vi "BallCacher.vi"() -> ()   [LabVIEW 2012]
doc: "This VI demonstrates how to control the Robotics Starter Kit 2.0 robot. It is deployed to an sbRIO-9632, then run on the Real-Time controller."
uses:
  <vilib>/Platform/TimedLoop/XDataNode/timing_clust.ctl
  <vilib>/Platform/TimedLoop/XDataNode/nitl_modes.ctl
  <vilib>/Platform/TimedLoop/XDataNode/wakeup.ctl
  <vilib>/robotics/Starter Kit/2.0/9632 Host Interface/NI_Robotics_Starter Kit Host_9632_2.0.lvclass
  <vilib>/Utility/AngleManip/Degrees to Radians (Scalar DBL).vi
  <vilib>/robotics/Steering/Steering Frame/Apply Steering Frame Velocity to Motors.vi
  <vilib>/Platform/TimedLoop/XDataNode/XDataNode.xnode
  <vilib>/Utility/AngleManip/NI_AngleManipulation.lvlib
  <vilib>/Platform/TimedLoop/XDataNode/XDNodeRunTimeDep.lvlib
  <vilib>/robotics/Utilities/Scan Angles/NI_Robotics_Scan Angles.lvlib
  <vilib>/robotics/Starter Kit/2.0/NI_Robotics_Starter Kit Host_2.0.lvlib
  <vilib>/robotics/Steering/Steering Frame/NI_Robotics_Steering Frame.lvclass
  <vilib>/robotics/Starter Kit/Host Interface/NI_Robotics_Starter Kit Host.lvclass
panel:
  in  "Tank1":dbl[](array[numeric])=[1.0, 1.0]
  in  "Tank2":dbl[](array[numeric])=[50.0, 50.0]
  out "Sensor Data":cluster{"angles (deg)":dbl[], "distances":dbl[]}(graph)
  in  "stop":bool
  # "This VI demonstrates how to control the Robotics Starter Kit 2.0 robot. It is deployed to an sbRIO-9632, then run on the Real-Time controller.\n\nInstructions:\n\n1. Set the \"MOTORS\" switch off, then set the \"MASTER\" switch on.  Make sure the robot is connected to the network.\n\n2. Run this VI.  The VI will deploy, and the robot's sensor will start panning left and right.  Accept any prompts to save VIs before deploying.\n\n3. Disconnect the robot from the network so it is no longer tethered.\n\n4. Move the robot to a clear area, then set the \"MOTORS\" switch on.  It will move and avoid obstacles.\n\n5. Set the \"MOTORS\" switch off to shut off power to the motors.\n\n6. Set the \"MASTER\" switch off to shut off power to the entire robot.  You will need to repeat steps 1 through 4 to redeploy after shutting off power*.\n\n*View Starter Kit 2.0 Readme.html for instructions on how to automatically run this VI on startup."
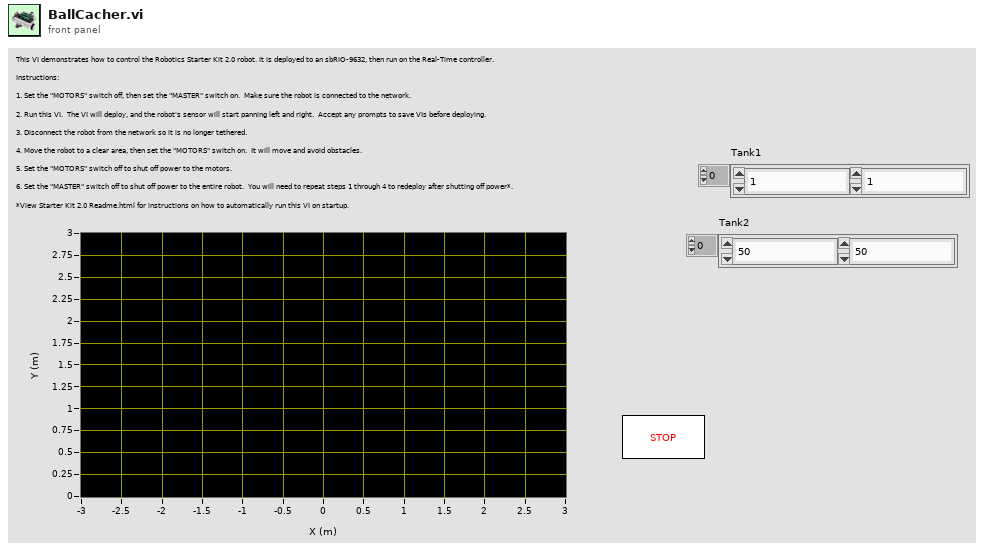
[diagram p1: front panel]
types:
  T1 = typedef "XDNodeRunTimeDep.lvlib/timing_clust.ctl" = cluster{"Expected End [f-1]":u64, "Actual End [f-1]":u64, "Finished Late? [f-1]":bool, "Expected End [i-1]":u64, "Actual End [i-1]":u64, "Finished Late? [i-1]":bool, "Expected Start [i]":u64, "Actual Start [i]":u64, "Expected Start [f]":u64, "Actual Start [f]":u64, "Source Name":string, "Structure Name":string, "Period":i64, "Deadline":i64, "Offset":i64, "Start":i64, "Priority":i32, "Timeout":i32, "Mode":T2, "Wakeup Reason":T3, "Error":errorcluster, "Source Type":string, "Secondary Source Type":string, "Global End Time":u64, "Global Start Time":u64, "Frame Duration":u64, "Iteration Duration":u64, "Assigned CPU":i32, "I/O Scan Engine Mode":u32}
  T2 = typedef "XDNodeRunTimeDep.lvlib/nitl_modes.ctl" = enum32{"No Change", "Process missed periods, maintain original phase", "Discard missed periods, maintain original phase", "Process missed periods, ignore original phase", "Discard missed periods, ignore original phase"}
  T3 = typedef "XDNodeRunTimeDep.lvlib/wakeup.ctl" = enum32{"Normal", "Aborted", "Asynchronous wakeup", "Timing source error", "Timed loop error", "Timeout"}
  T4 = typedef "NI_Robotics_Scan Angles.lvlib/Scan Angle Data.ctl" = cluster{"angles":dbl[], "distances":dbl[], "current index":i32, "previous index":i32}
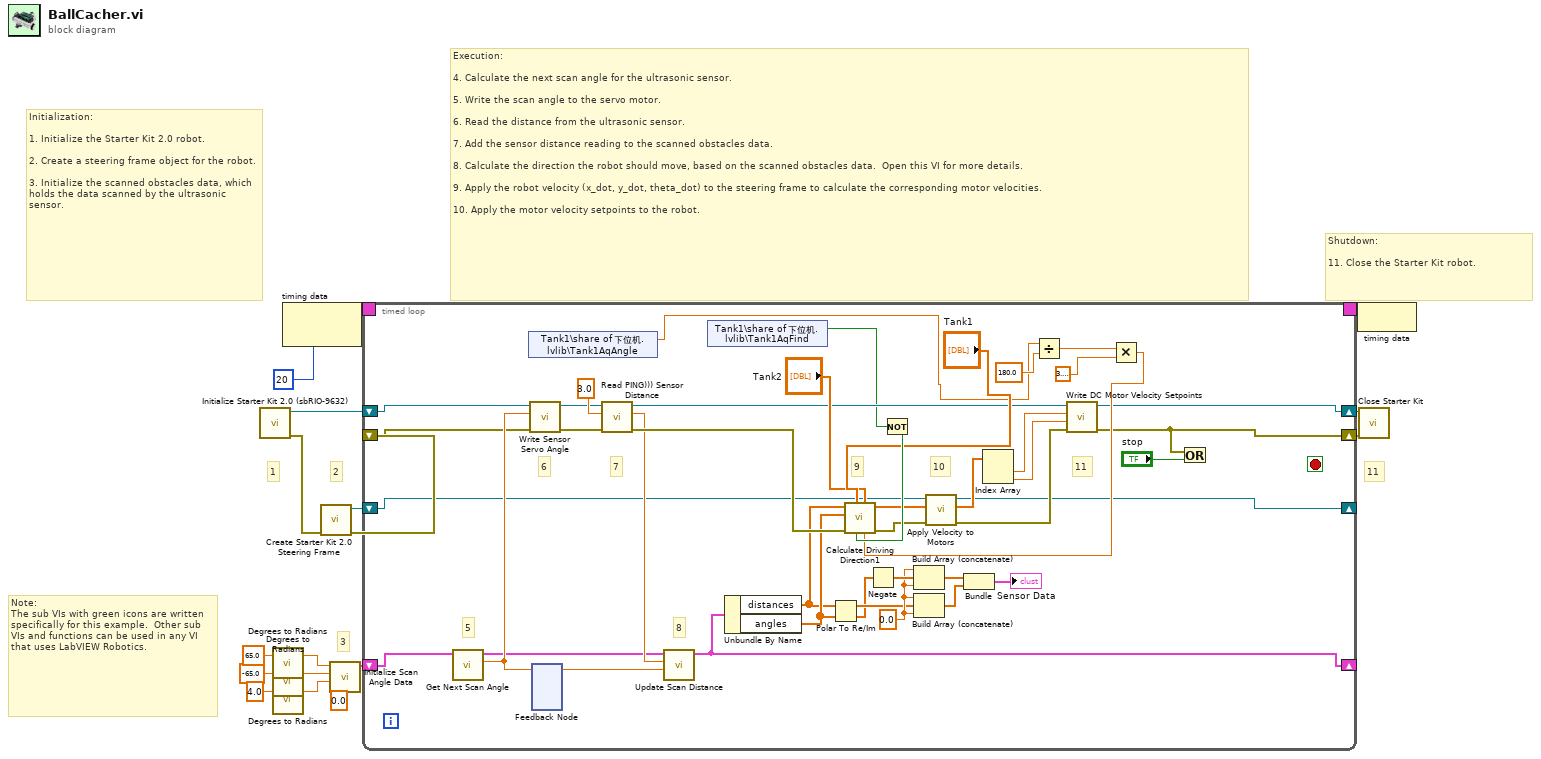
[diagram p0: block diagram]
diagram:
  # "11"
  # "Shutdown:\n\n11. Close the Starter Kit robot."
  # "Execution:\n\n4. Calculate the next scan angle for the ultrasonic sensor.\n\n5. Write the scan angle to the servo motor.\n\n6. Read the distance from the ultrasonic sensor.\n\n7. Add the sensor distance reading to the scanned obstacles data.\n\n8. Calculate the direction the robot should move, based on the scanned obstacles data.  Open this VI for more details.\n\n9. Apply the robot velocity (x_dot, y_dot, theta_dot) to the steering frame to calculate the corresponding motor velocities.\n\n10. Apply the motor velocity setpoints to the robot."
  # "3"
  # "2"
  # "1"
  # "Initialization:\n\n1. Initialize the Starter Kit 2.0 robot.\n\n2. Create a steering frame object for the robot.\n\n3. Initialize the scanned obstacles data, which holds the data scanned by the ultrasonic sensor."
  # "Note:\nThe sub VIs with green icons are written specifically for this example.  Other sub VIs and functions can be used in any VI that uses LabVIEW Robotics."
  n1 = call <vilib>:"Initialize Starter Kit 2.0 (sbRIO-9632).vi"() -> ("error out"=w1:errorcluster, "FPGA starter kit host 2.0 out"=w2:refnum<class "NI_Robotics_Starter Kit Host_9632_2.0.lvclass">)  [unwired: 10 in]
  n2 = call-poly <vilib>:"Degrees to Radians.vi"("angle (deg)"=65.0 ("max angle")) -> ("angle (rad)"=w12:dbl)  [unwired: 2 in]
  n3 = call-poly <vilib>:"Degrees to Radians.vi"("angle (deg)"=-65.0 ("min angle")) -> ("angle (rad)"=w8:dbl)  [unwired: 2 in]
  n4 = call-poly <vilib>:"Degrees to Radians.vi"("angle (deg)"=4.0 ("scan angle")) -> ("angle (rad)"=w9:dbl)  [unwired: 2 in]
  n5 = node-c288(i64 20 ("Period")) -> (w17:T1)
  n6 = call <vilib>:"Create Starter Kit 2.0 Steering Frame.vi"("error in (no error)"=w1) -> ("error out"=w5:errorcluster, "starter kit differential steering frame"=w6:refnum<class "NI_Robotics_Differential Steering Frame.lvclass">)  [unwired: 9 in]
  n7 = call <vilib>:"Initialize Scan Angle Data.vi"("initial angle (0)"=0.0, "scan angle"=w9, "min angle"=w8, "max angle"=w12) -> ("scan angles"=w14:T4)  [unwired: 6 in, 1 out]
  n8 = timed-loop {
    shift-right: [w20] -> _
    shift-left: w14 -> [w27]
    timing: w17 -> [_]
    timing-out: [_] -> w16
    shift-right: [w22] -> w3
    shift-left: w5 -> [w25]
    shift-right: [w23] -> w4
    shift-left: w2 -> [w24]
    shift-right: [w21] -> _
    shift-left: w6 -> [w26]
    stop <- _ stop-if-true
    w44 = 0.0 ("element")
    # "7"
    # "6"
    # "11"
    # "10"
    # "9"
    # "8"
    # "5"
    n9 = call <vilib>:"Get Next Scan Angle.vi"("scan angles in"=w27) -> ("new angle"=w32:dbl, "scan angles out"=w29:T4)  [unwired: 9 in]
    n10 = shared-variable "Tank1\\share of 下位机.lvlib\\Tank1AqAngle"() -> (w18:dbl)  [unwired: 1 in, 1 out]
    n11 = call <vilib>:"Write Sensor Servo Angle.vi"("error in (no error)"=w25, "ccw servo angle (rad)"=w32, "starter kit host in"=w24) -> ("error out"=w35:errorcluster, "starter kit host out"=w34:refnum<class "NI_Robotics_Starter Kit Host_9632_2.0.lvclass">)  [unwired: 7 in]
    n12 = feedback #1() -> (w30:dbl)  [unwired: 1 in]
    n13 = feedback-in #1(w32) -> ()
    n14 = call <vilib>:"Read PING))) Sensor Distance.vi"("error in (no error)"=w35, "default distance (NaN)"=3.0, "starter kit host in"=w34) -> ("error out"=w51:errorcluster, "distance (m)"=w33:dbl, "starter kit host out"=w36:refnum<class "NI_Robotics_Starter Kit Host_9632_2.0.lvclass">)  [unwired: 5 in, 1 out]
    n15 = call <vilib>:"Update Scan Distance.vi"("scan angle"=w30, "new scan distance"=w33, "scan angles in"=w29) -> ("scan angles out"=w20:T4)  [unwired: 8 in]
    n16 = shared-variable "Tank1\\share of 下位机.lvlib\\Tank1AqFind"() -> (w19:bool)  [unwired: 1 in, 1 out]
    n17 = Unbundle By Name(w20) -> ("distances"=w48:dbl[], "angles"=w50:dbl[])
    n18 = Polar To Re/Im(2:w50, 3:w48) -> (0:w41:dbl[], 1:w42:dbl[])
    n19 = Negate(x=w41) -> (-x=w46:dbl[])
    n20 = Not(x=w19) -> (.not. x?=w59:bool)
    n21 = Build Array (concatenate)(w44, w46, w44) -> (w45:dbl[])
    n22 = Build Array (concatenate)(w44, w42, w44) -> (w43:dbl[])
    n23 = Bundle(w45, w43) -> (→"Sensor Data":cluster{dbl[], dbl[]})  [unwired: 1 in]
    n24 = Divide(x=w18, y=180.0 ("initial angle (0)")) -> (x/y=w54:dbl)
    n25 = Multiply(x=w54, y=3.141592653589793) -> (x*y=w58:dbl)
    n26 = call "Calculate Driving Direction1.vi"("angle"=w58, "Tank2"="Tank2", "Identity"=w59, "Tank1"="Tank1", "error in (no error)"=w51, "obstacle angles (rad)"=w50, "obstacle distances (m)"=w48) -> ("error out"=w52:errorcluster, "steering frame velocity"=w49:dbl[])  [unwired: 3 in]
    n27 = call-poly <vilib>:"Apply Velocity to Motors.vi"("error in (no error)"=w52, "steering frame velocity"=w49, "steering frame in"=w26) -> ("error out"=w37:errorcluster, "ccw motor velocity setpoints"=w31:dbl[], "steering frame out"=w21:refnum<class "NI_Robotics_Differential Steering Frame.lvclass">)  [unwired: 4 in, 2 out]
    n28 = Index Array(array=w31) -> (element #1=w38:dbl, element #2=w39:dbl)  [unwired: 2 in]
    n29 = call <vilib>:"Write DC Motor Velocity Setpoints.vi"("error in (no error)"=w37, "right motor ccw velocity (rad/s)"=w39, "left motor ccw velocity (rad/s)"=w38, "starter kit host in"=w36) -> ("error out"=w22:errorcluster, "starter kit host out"=w23:refnum<class "NI_Robotics_Starter Kit Host_9632_2.0.lvclass">)  [unwired: 6 in]
    n30 = Or(x=w22, y="stop") -> ()  [unwired: 1 out]
  }
  n31 = node-c288(w16) -> ()
  n32 = call-dynamic "Close Starter Kit.vi"("error in (no error)"=w3, "starter kit host in"=w4) -> ()  [unwired: 9 in, 1 out]
